vi "Agilent 681x Standard Configured Output.vi"() -> ()   [LabVIEW 2019]
doc: "Shows how to generate a standard output."
uses:
  <instrlib>/Agilent 681x Series/Agilent 681x Series.lvlib
panel:
  in  "Peak Current Limit (13 A)":dbl=13.0 format="%#.4g"
  in  "RMS Current Limit (1 A)":dbl=1.0 format="%#.4g"
  in  "Voltage Amplitude (1.0 V)":dbl=1.0 format="%#.4g"
  in  "Output Frequency (60 Hz)":dbl=60.0 format="%#.4g"
  in  "Output Waveform Type (0: Sinusoid)":u16(ring) items=["Sinusoid", "Square", "Clipped Sinusoid", "User Specified"]
  in  "User-Specified Output Waveform Name":string
  in  "Serial Configuration":T1={"Baud Rate"=9600, "Parity"=0, "Data Bits"=7} {"Data Bits" items=["7"=7, "8"=8]; "Parity" items=["None", "Odd", "Even", "Mark", "Space"]; "Baud Rate" items=["300"=300, "600"=600, "1200"=1200, "2400"=2400, "4800"=4800, "9600"=9600]}
  in  "VISA resource name":refnum<visa-resource-name>
  # "(c) 2008-2021 National Instruments Corp.  ALL RIGHTS RESERVED."
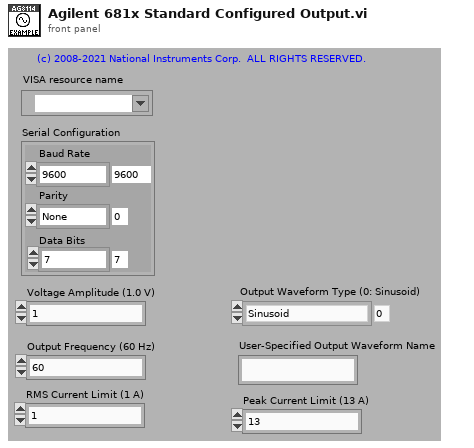
[diagram p1: front panel]
types:
  T1 = cluster{"Baud Rate":u32, "Parity":u16, "Data Bits":u16}
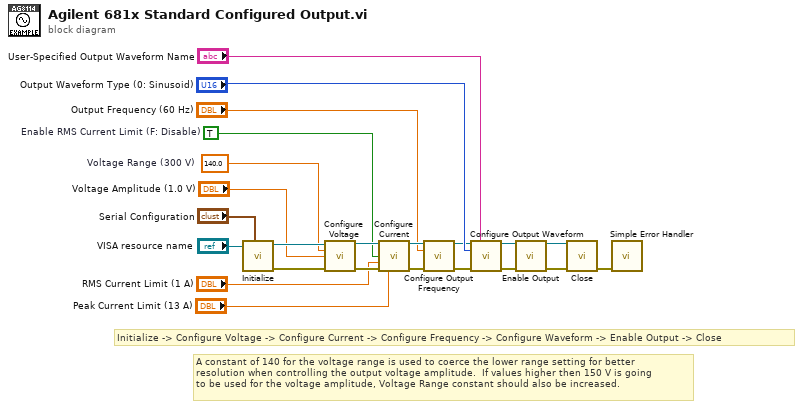
[diagram p0: block diagram]
diagram:
  w9 = TRUE  # Enable RMS Current Limit (F: Disable)
  w16 = 140.0  # Voltage Range (300 V)
  # "Initialize -> Configure Voltage -> Configure Current -> Configure Frequency -> Configure Waveform -> Enable Output -> Close"
  # "A constant of 140 for the voltage range is used to coerce the lower range setting for better\nresolution when controlling the output voltage amplitude.  If values higher then 150 V is going\nto be used for the voltage amplitude, Voltage Range constant should also be increased."
  n1 = call <instrlib>:"Initialize.vi"("Serial Configuration"="Serial Configuration", "VISA resource name"="VISA resource name") -> ("error out"=w20:errorcluster, "VISA resource name out"=w21:refnum<visa-resource-name>)  [unwired: 8 in]
  n2 = call <instrlib>:"Configure Voltage.vi"("VISA resource name"=w21, "Voltage Range (300 V)"=w16, "Voltage Amplitude (1.0 V)"="Voltage Amplitude (1.0 V)", "error in (no error)"=w20) -> ("VISA resource name out"=w19:refnum<visa-resource-name>, "error out"=w18:errorcluster)  [unwired: 10 in]
  n3 = call <instrlib>:"Configure Current.vi"("VISA resource name"=w19, "Enable RMS Current Limit (F: Disable)"=w9, "RMS Current Limit (1 A)"="RMS Current Limit (1 A)", "error in (no error)"=w18, "Peak Current Limit (13 A)"="Peak Current Limit (13 A)") -> ("VISA resource name out"=w12:refnum<visa-resource-name>, "error out"=w13:errorcluster)  [unwired: 9 in]
  n4 = call <instrlib>:"Configure Output Frequency.vi"("VISA resource name"=w12, "Output Frequency (60 Hz)"="Output Frequency (60 Hz)", "error in (no error)"=w13) -> ("VISA resource name out"=w10:refnum<visa-resource-name>, "error out"=w11:errorcluster)  [unwired: 11 in]
  n5 = call <instrlib>:"Configure Output Waveform.vi"("VISA resource name"=w10, "User-Specified Output Waveform Name"="User-Specified Output Waveform Name", "Output Waveform Type (0: Sinusoid)"="Output Waveform Type (0: Sinusoid)", "error in (no error)"=w11) -> ("VISA resource name out"=w14:refnum<visa-resource-name>, "error out"=w15:errorcluster)  [unwired: 10 in]
  n6 = call <instrlib>:"Enable Output.vi"("VISA resource name"=w14, "error in (no error)"=w15) -> ("VISA resource name out"=w6:refnum<visa-resource-name>, "error out"=w7:errorcluster)  [unwired: 12 in]
  n7 = call <instrlib>:"Close.vi"("error in (no error)"=w7, "VISA resource name"=w6) -> ("error out"=w5:errorcluster)  [unwired: 9 in]
  n8 = call <vilib>:"Simple Error Handler.vi"("error in (no error)"=w5) -> ()  [unwired: 4 in, 5 out]
